vi "FR GUI Measurement setup.vi"(7 "Common properties":T1={"Measurement status ref"=refnum, "TWM Status ref"=refnum, "Abort ref"=refnum, "Skip waiting ref"=refnum, "GNU Octave path"=path "C:/Program Files/GNU Octave/Octave-6.2.0/mingw64/bin", "TWM+QWTB path"=path "C:/Users/labina/Desktop/TWM-1.8.7.0-full/octprog", "lvlib path"=path "D:/martin/WAC/WACsw - github/control_software/Filter function meter/external libraries/GOLPI 0.7.3.1 source distribution LV 20.0 32 bit/lv_proc.dll", "TWM pipe"="\\\\.\\pipe\\TWM:server", "PJVS status ref"=refnum, "WAC path"=path ""}, 8 "DC meter":T2={"DC meter type"=enum."H/A/K 3458", "DC meter VISA"="", "NPLC"=10.0, "status ref"=refnum}, 9 "FR measurement":T4={"Measurement frequencies (Hz)"=[1000.0, 10000.0, 1000.0], "Sampling frequency (Hz)"=500000.0, "Signal amplitude (V)"=4.5, "AC-DC settle time (s)"=20.0, "Record length (multiples of period)"=[1000.0, 10000.0, 1000.0], "Measurement template file"=path "", "Row of START keyword"=0, "Row of STOP keyword"=0, "Calculate RMS from samples"=FALSE, "AC-DC warm up time (s)"=300.0, "Measurement template line"=[], "DC meter readings No."=10, "Algorithm"="TWM-WFFT", "Simultaneous measurement"=FALSE, "Recalculate-skip already calculated"=FALSE} {"Record length (multiples of period)" format="%#_3p"; "Sampling frequency (Hz)" format="%#_3p"; "Measurement frequencies (Hz)" format="%#_3p"}) -> (1 "Common properties out":T1={"Measurement status ref"=refnum, "TWM Status ref"=refnum, "Abort ref"=refnum, "Skip waiting ref"=refnum, "GNU Octave path"=path "C:/Program Files/GNU Octave/Octave-6.2.0/mingw64/bin", "TWM+QWTB path"=path "C:/Users/labina/Desktop/TWM-1.8.7.0-full/octprog", "lvlib path"=path "D:/martin/WAC/WACsw - github/control_software/Filter function meter/external libraries/GOLPI 0.7.3.1 source distribution LV 20.0 32 bit/lv_proc.dll", "TWM pipe"="\\\\.\\pipe\\TWM:server", "PJVS status ref"=refnum, "WAC path"=path ""}, 3 "FR measurement out":T4={"Measurement frequencies (Hz)"=[1000.0, 10000.0, 1000.0], "Sampling frequency (Hz)"=500000.0, "Signal amplitude (V)"=4.5, "AC-DC settle time (s)"=20.0, "Record length (multiples of period)"=[1000.0, 10000.0, 1000.0], "Measurement template file"=path "", "Row of START keyword"=0, "Row of STOP keyword"=0, "Calculate RMS from samples"=FALSE, "AC-DC warm up time (s)"=300.0, "Measurement template line"=[], "DC meter readings No."=10, "Algorithm"="TWM-WFFT", "Simultaneous measurement"=FALSE, "Recalculate-skip already calculated"=FALSE} {"Record length (multiples of period)" format="%#_3p"; "Sampling frequency (Hz)" format="%#_3p"; "Measurement frequencies (Hz)" format="%#_3p"})   [LabVIEW 2020]
doc: "GUI to setup parameters of the mesurement procedure used to estimate frequency response of the digitizer."
uses:
  FR Measurement/Type definitions/FR measuement.ctl
  General DC meter/Type definitions/DC meter.ctl
  General DC meter/Type definitions/DC meter type.ctl
  Utilities/Type definitions/Common properties.ctl
  <vilib>/Utility/error.llb/Error Cluster From Error Code.vi
  <vilib>/ErrorRing/Error Ring.xnode
  external libraries/varilib/varilib.lvlib
panel:
  out "Simultaneous\nmeasurement":bool
  out "Algorithm":string
  out "dc meter readings":i32=50000 caption="DC meter readings"
  in  "recalculate template":bool
  out "ac-dc warmup time":dbl=50000.0 caption="AC-DC warm-up time" format="%#_6p"
  out "Estimate as formatted text":string
  out "Meas points":i32=1 caption="Measurement points"
  in  "Calculate RMS\nfrom samples":bool
  out "ac-dc settle time":dbl=50000.0 caption="AC-DC settle time" format="%#_6p"
  out "Measurement freq. (Hz) | Record length (periods)":dbl[][](array[numeric])=[[1000.0]] format="%#_3p"
  in  "load template":bool
  in  "Measurement template file":path
  in  "show connections":bool
  out "Signal amplitude (V)":dbl=1.0 caption="AC voltage amplitude"
  out "Sampling frequency (Hz)":dbl=50000.0 caption="Sampling frequency" format="%#_6p"
  out "gui_elements":refnum<vi>[](array[refnum])
  in  "save_and_quit":bool
  in  "cancel":bool
  # "Load the template and check loaded values here:"
  # "s"
  # "V"
  # "Who will make\nnice pictures?\n\nconnection setup here"
  # "Hz"
  # "s"
  # "Who will make\nnice pictures?\n\nwaveforms here"
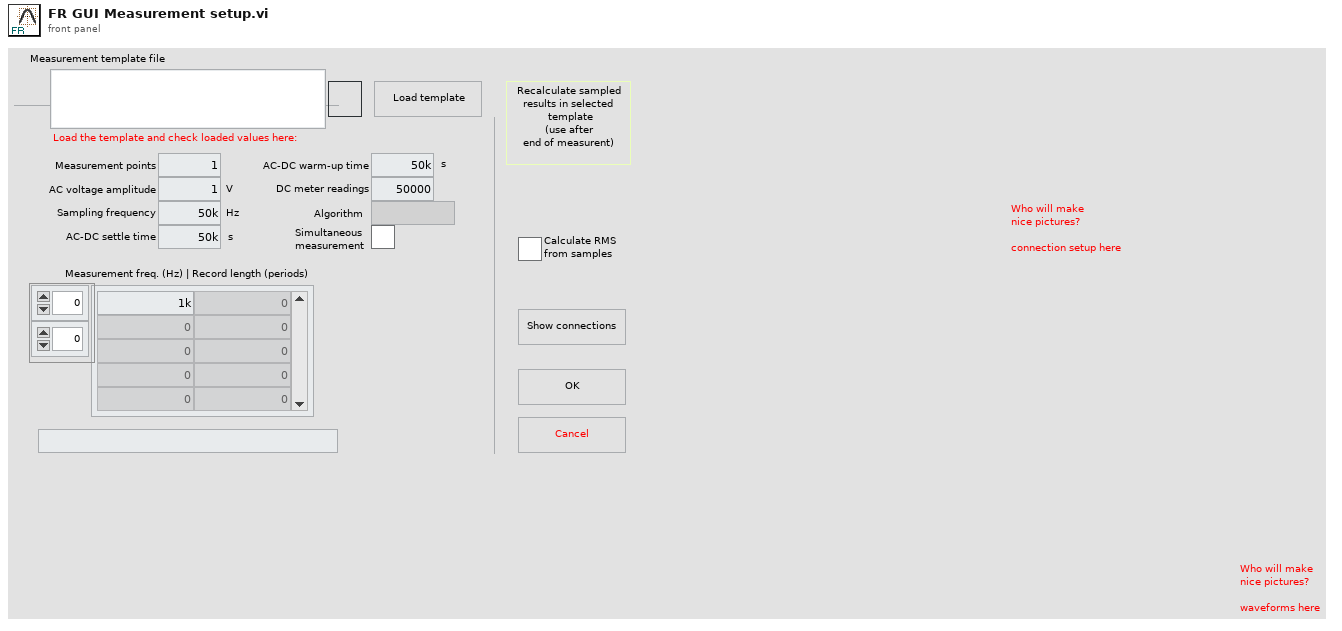
[diagram p1: front panel]
types:
  T1 = typedef "Common properties.ctl" = cluster{"Measurement status ref":refnum<vi>, "TWM Status ref":refnum<vi>, "Abort ref":refnum<vi>, "Skip waiting ref":refnum<vi>, "GNU Octave path":path, "TWM+QWTB path":path, "lvlib path":path, "TWM pipe":string, "PJVS status ref":refnum<vi>, "WAC path":path}
  T2 = typedef "DC meter.ctl" = cluster{"DC meter type":T3, "DC meter VISA":refnum<visa-resource-name>, "NPLC":dbl, "status ref":refnum<vi>}
  T3 = typedef "DC meter type.ctl" = enum16{"H/A/K 3458", "Fluke 8508A", "dummy", "Keithley 2182"}
  T4 = typedef "FR measuement.ctl" = cluster{"Measurement frequencies (Hz)":dbl[], "Sampling frequency (Hz)":dbl, "Signal amplitude (V)":dbl, "AC-DC settle time (s)":dbl, "Record length (multiples of period)":dbl[], "Measurement template file":path, "Row of START keyword":i32, "Row of STOP keyword":i32, "Calculate RMS from samples":bool, "AC-DC warm up time (s)":dbl, "Measurement template line":i32[], "DC meter readings No.":i32, "Algorithm":string, "Simultaneous measurement":bool, "Recalculate-skip already calculated":bool}
  T5 = enum32{"Bad", "Idle", "Run top level", "Running"}
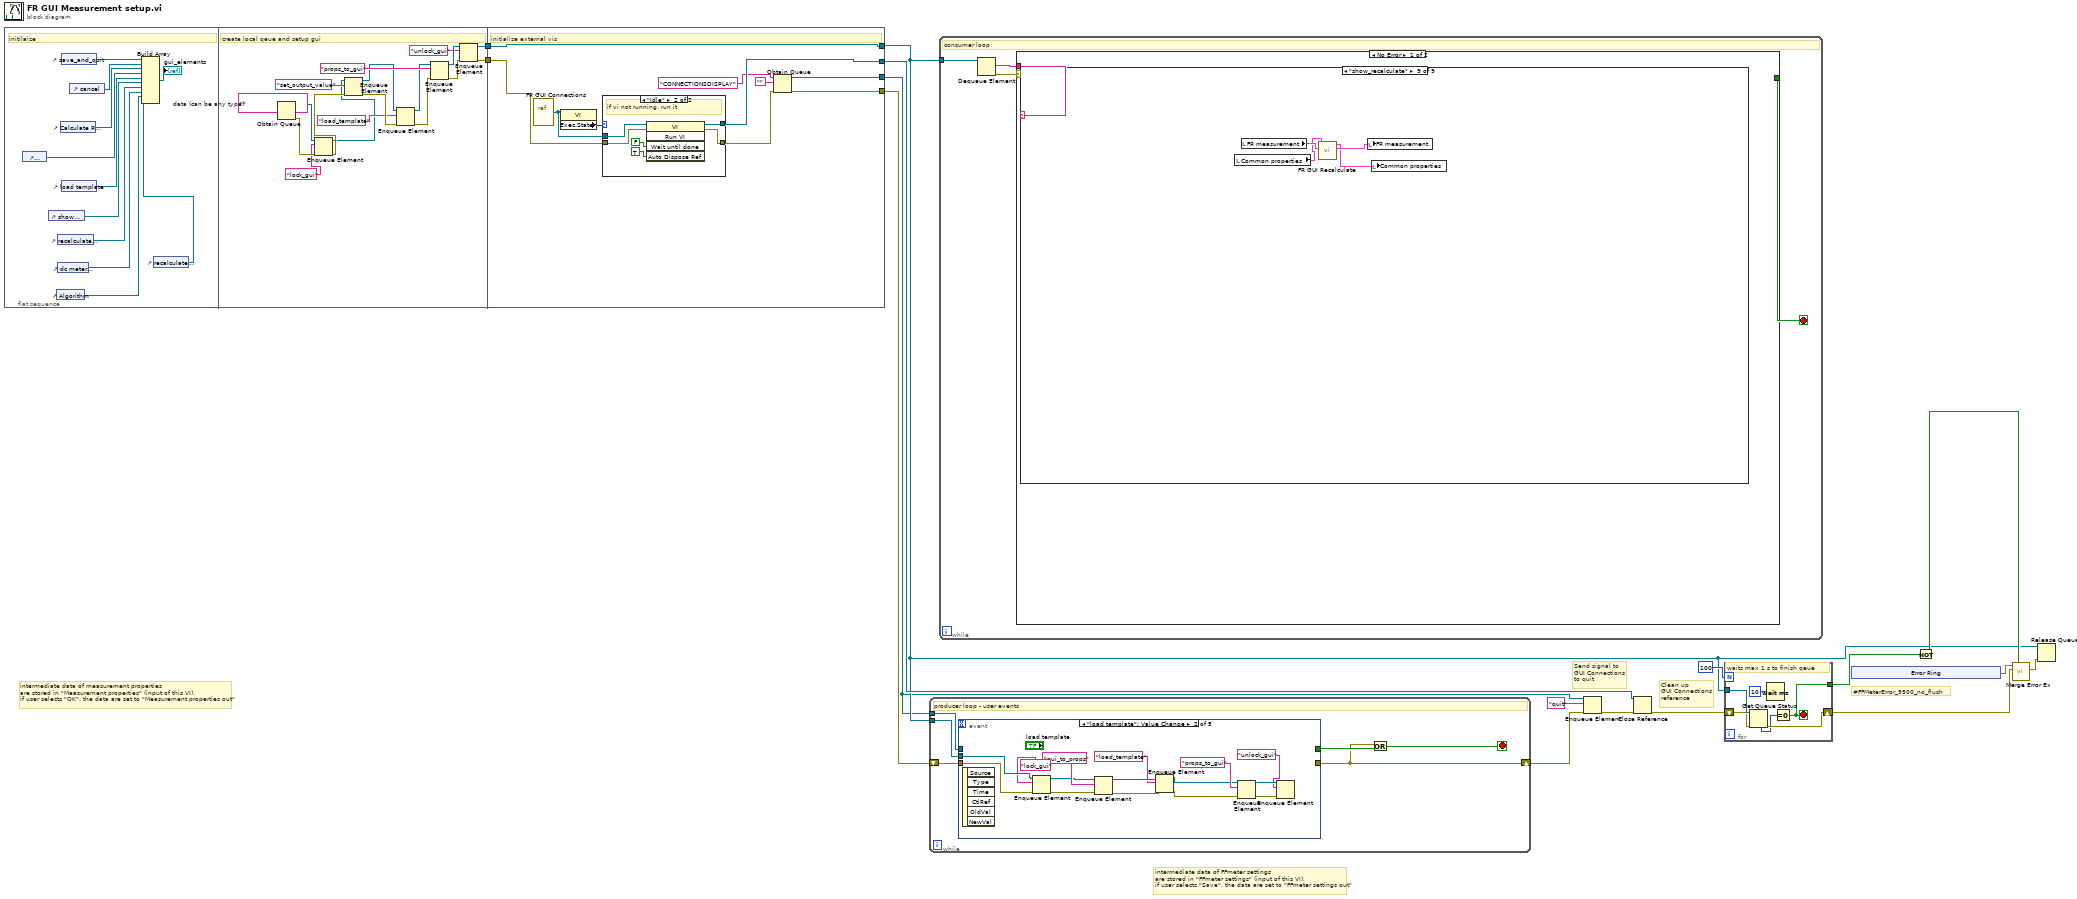
[diagram p0: block diagram]
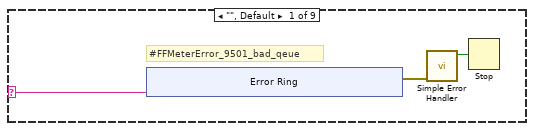
[diagram p3: hidden frame]
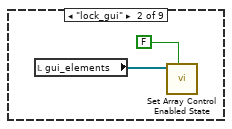
[diagram p4: hidden frame]
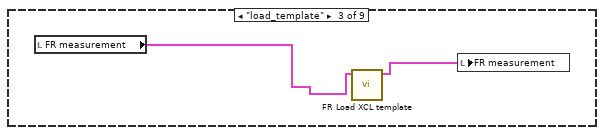
[diagram p5: hidden frame]
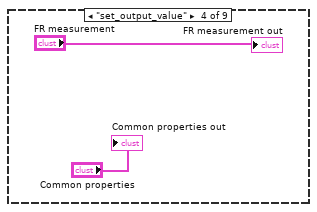
[diagram p6: hidden frame]
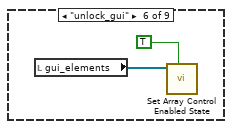
[diagram p8: hidden frame]
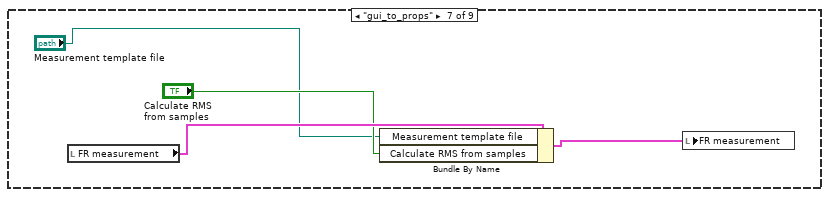
[diagram p9: hidden frame]
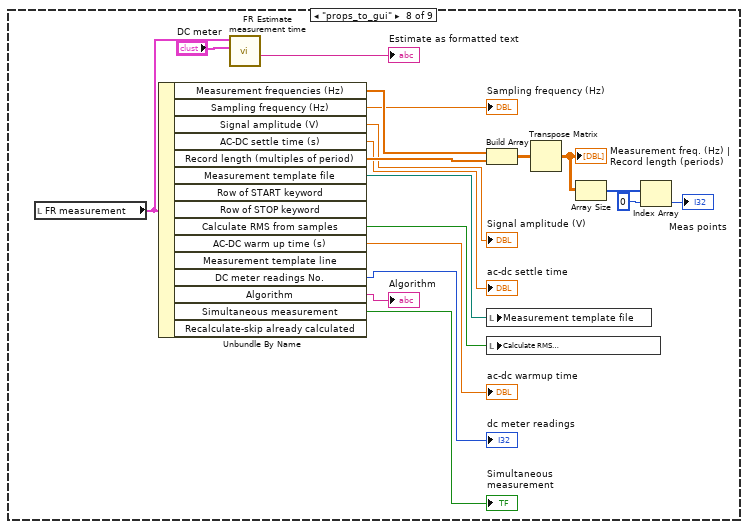
[diagram p10: hidden frame]
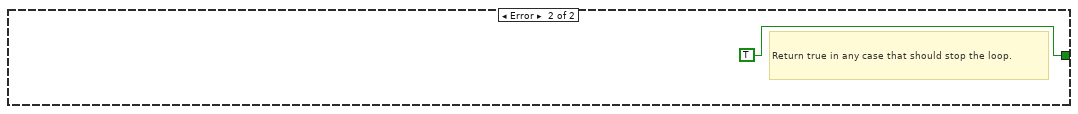
[diagram p11: hidden frame]
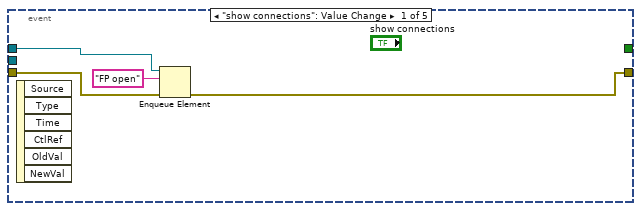
[diagram p12: hidden frame]
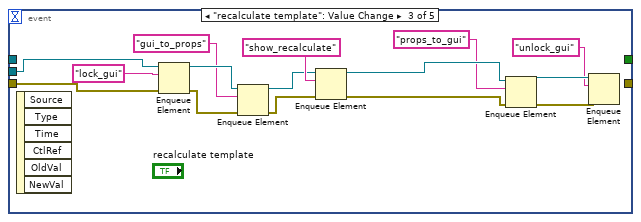
[diagram p13: hidden frame]
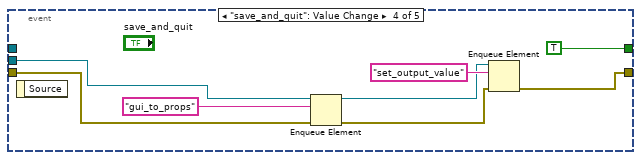
[diagram p14: hidden frame]
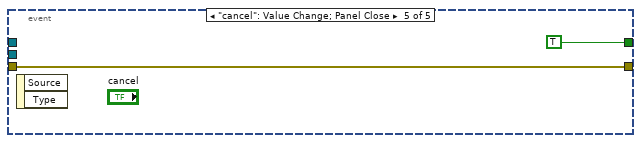
[diagram p15: hidden frame]
diagram:
  # "intermediate data of measurement properties\nare stored in \"Measurement properties\" (input of this VI),\nif user selects \"OK\", the data are set to \"Measurement properties out\""
  # "intermediate data of FFmeter settings\nare stored in \"FFmeter settings\" (input of this VI),\nif user selects \"Save\", the data are set to \"FFmeter settings out\""
  # "Send signal to\nGUI Connections\nto quit"
  # "Clean up\nGUI Connections\nreference"
  # "#FFMeterError_9500_no_flush"
  n1 = flat-sequence {
    tunnel: [w41] -> w9
    tunnel: [w42] -> w8
    tunnel: [w51] -> w10
    tunnel: [w55] -> w3
    tunnel: w9 -> [w55]
    tunnel: w8 -> [w54]
    tunnel: [w52] -> w2
    tunnel: [w53] -> w5
    frame #0 {
      # "initilaize"
      n2 = control-ref of="Measurement template file"() -> (w23:refnum<vi>)
      n3 = control-ref of="show connections"() -> (w21:refnum<vi>)
      n4 = control-ref of="Algorithm"() -> (w18:refnum<vi>)
      n5 = control-ref of="dc meter readings"() -> (w19:refnum<vi>)
      n6 = control-ref of="recalculate template"() -> (w20:refnum<vi>)
      n7 = control-ref of="Calculate RMS\nfrom samples"() -> (w24:refnum<vi>)
      n8 = control-ref of="save_and_quit"() -> (w27:refnum<vi>)
      n9 = control-ref of="load template"() -> (w22:refnum<vi>)
      n10 = control-ref of="cancel"() -> (w26:refnum<vi>)
      n11 = control-ref of="recalculate template"() -> (w17:refnum<vi>)
      n12 = Build Array(w27, w26, w24, w23, w22, w21, w20, w19, w18, w17) -> (→"gui_elements":refnum<vi>[])
    }
    frame #1 {
      w44 = ""  # data (can be any type)
      # "create local qeue and setup gui"
      n13 = Obtain Queue(element data type=w44) -> (queue out=w29:refnum<queue>, error out=w32:errorcluster)  [unwired: 4 in, 1 out]
      n14 = Enqueue Element(queue=w29, element="lock_gui", error in (no error)=w32) -> (queue out=w30:refnum<queue>, error out=w31:errorcluster)  [unwired: 1 in, 1 out]
      n15 = Enqueue Element(queue=w30, element="set_output_value", error in (no error)=w31) -> (queue out=w35:refnum<queue>, error out=w37:errorcluster)  [unwired: 1 in, 1 out]
      n16 = Enqueue Element(queue=w35, element="load_template", error in (no error)=w37) -> (queue out=w34:refnum<queue>, error out=w36:errorcluster)  [unwired: 1 in, 1 out]
      n17 = Enqueue Element(queue=w34, element="props_to_gui", error in (no error)=w36) -> (queue out=w40:refnum<queue>, error out=w43:errorcluster)  [unwired: 1 in, 1 out]
      n18 = Enqueue Element(queue=w40, element="unlock_gui", error in (no error)=w43) -> (queue out=w41:refnum<queue>, error out=w42:errorcluster)  [unwired: 1 in, 1 out]
    }
    frame #2 {
      # "initialize external vis"
      n19 = vi-ref "FR GUI Connections.vi"() -> (w49:refnum<vi>)
      n20 = property class="VI"(reference=w49) -> ("Exec.State"=w50:T5)  [unwired: 1 in, 2 out]
      n21 = case shown="\"Idle\"" w50 {
        tunnel: [w56 w63] -> w46
        tunnel: w54 -> [w56 w60]
        tunnel: [w57 w59] -> w53
        tunnel: w49 -> [w57 w58]
        frame "Bad", Default {
        }
        frame "Idle" {
          # "if vi not running, run it"
          n22 = invoke class="VI" method="Run VI"(reference=w58, error in=w60, "Wait until done"=FALSE ("Wait Until Done"), "Auto Dispose Ref"=TRUE ("Wait Until Done")) -> (reference out=w59:refnum<vi>, error out=w63:errorcluster)  [unwired: 1 in, 3 out]
        }
      }
      n23 = Obtain Queue(name (unnamed)="CONNECTIONSDISPLAY", element data type="", error in (no error)=w46) -> (queue out=w52:refnum<queue>, error out=w51:errorcluster)  [unwired: 2 in, 1 out]
    }
  }
  n24 = while {
    shift-right: [w65] -> w4
    shift-left: w10 -> [w68]
    tunnel: w3 -> [w69]
    tunnel: w2 -> [w64]
    stop <- w66 stop-if-true
    # "producer loop - user events"
    n25 = event shown="[1] \"load template\": Value Change" {
      selector: _ -> [_ _ _ _ _]
      dyn-events: _ -> [_ _ _ _ _]
      timeout: _ -> [_ _ _ _ _]
      tunnel: w69 -> [_ w78 w98 w110 _]
      tunnel: w68 -> [w72 w75 w99 w109 w112]
      tunnel: [w71 _ _ w107 w112] -> w65
      tunnel: [_ _ _ TRUE ("cancel") TRUE ("cancel")] -> w67
      tunnel: w64 -> [w70 _ _ _ _]
      event "show connections": Value Change {
        n26 = event-data() -> ()  [unwired: 1 in, 6 out]
        n27 = Enqueue Element(queue=w70, element="FP open", error in (no error)=w72) -> (error out=w71:errorcluster)  [unwired: 1 in, 2 out]
      }
      event "load template": Value Change {
        n28 = event-data() -> ()  [unwired: 1 in, 6 out]
        n29 = Enqueue Element(queue=w78, element="lock_gui", error in (no error)=w75) -> (queue out=w77:refnum<queue>, error out=w76:errorcluster)  [unwired: 1 in, 1 out]
        n30 = Enqueue Element(queue=w77, element="gui_to_props", error in (no error)=w76) -> (queue out=w84:refnum<queue>, error out=w86:errorcluster)  [unwired: 1 in, 1 out]
        n31 = Enqueue Element(queue=w84, element="load_template", error in (no error)=w86) -> (queue out=w83:refnum<queue>, error out=w85:errorcluster)  [unwired: 1 in, 1 out]
        n32 = Enqueue Element(queue=w83, element="props_to_gui", error in (no error)=w85) -> (queue out=w80:refnum<queue>, error out=w81:errorcluster)  [unwired: 1 in, 1 out]
        n33 = Enqueue Element(queue=w80, element="unlock_gui", error in (no error)=w81) -> ()  [unwired: 1 in, 3 out]
      }
      event "recalculate template": Value Change {
        n34 = event-data() -> ()  [unwired: 1 in, 6 out]
        n35 = Enqueue Element(queue=w98, element="lock_gui", error in (no error)=w99) -> (queue out=w93:refnum<queue>, error out=w96:errorcluster)  [unwired: 1 in, 1 out]
        n36 = Enqueue Element(queue=w93, element="gui_to_props", error in (no error)=w96) -> (queue out=w94:refnum<queue>, error out=w95:errorcluster)  [unwired: 1 in, 1 out]
        n37 = Enqueue Element(queue=w94, element="show_recalculate", error in (no error)=w95) -> (queue out=w101:refnum<queue>, error out=w102:errorcluster)  [unwired: 1 in, 1 out]
        n38 = Enqueue Element(queue=w101, element="props_to_gui", error in (no error)=w102) -> (queue out=w90:refnum<queue>, error out=w91:errorcluster)  [unwired: 1 in, 1 out]
        n39 = Enqueue Element(queue=w90, element="unlock_gui", error in (no error)=w91) -> ()  [unwired: 1 in, 3 out]
      }
      event "save_and_quit": Value Change {
        n40 = event-data() -> ()  [unwired: 1 in, 1 out]
        n41 = Enqueue Element(queue=w110, element="gui_to_props", error in (no error)=w109) -> (queue out=w104:refnum<queue>, error out=w108:errorcluster)  [unwired: 1 in, 1 out]
        n42 = Enqueue Element(queue=w104, element="set_output_value", error in (no error)=w108) -> (error out=w107:errorcluster)  [unwired: 1 in, 2 out]
      }
      event "cancel": Value Change; Panel Close {
        n43 = event-data() -> ()  [unwired: 1 in, 2 out]
      }
    }
    n44 = Or(x=w65, y=w67) -> (x .or. y?=w66:bool)
  }
  n45 = while {
    tunnel: w3 -> [w117]
    stop <- w114 stop-if-true
    # "consumer loop"
    n46 = Dequeue Element(queue=w117) -> (element=w115:string, error out=w116:errorcluster)  [unwired: 2 in, 2 out]
    n47 = case shown="No Error" w116 {
      tunnel: w115 -> [w118 _]
      tunnel: [_ TRUE] -> w114
      frame No Error {
        n48 = case shown="\"show_recalculate\"" w118 {
          selector: w118 -> [w119 _ _ _ _ _ _ _ _]
          frame "", Default {
            # "#FFMeterError_9501_bad_qeue"
            n49 = xnode "Error Ring"("parameter 0"=w119) -> ("error out"=w121:errorcluster)
            n50 = call <vilib>:"Simple Error Handler.vi"("error in (no error)"=w121) -> ("error?"=w120:bool)  [unwired: 4 in, 4 out]
            n51 = Stop(stop? (T)=w120) -> ()
          }
          frame "lock_gui" {
            n52 = local read "gui_elements"() -> (w130:refnum<vi>[])
            n53 = call "Set Array Control Enabled State.vi"("enabled (T)"=FALSE, "reference array in"=w130) -> ()  [unwired: 8 in, 2 out]
          }
          frame "load_template" {
            n54 = local read "FR measurement"() -> (w131:T4)
            n55 = call "FR Load XCL template.vi"("FR measurement"=w131) -> ("FR measurement out"=w132:T4)  [unwired: 10 in]
            n56 = local write "FR measurement"(w132) -> ()
          }
          frame "set_output_value" {
            "FR measurement out" <- "FR measurement"
            "Common properties out" <- "Common properties"
          }
          frame "create_template" {
          }
          frame "unlock_gui" {
            n57 = local read "gui_elements"() -> (w136:refnum<vi>[])
            n58 = call "Set Array Control Enabled State.vi"("enabled (T)"=TRUE, "reference array in"=w136) -> ()  [unwired: 8 in, 2 out]
          }
          frame "gui_to_props" {
            n59 = local read "FR measurement"() -> (w140:T4)
            n60 = Bundle By Name(cluster=w140, "Measurement template file"="Measurement template file", "Calculate RMS from samples"="Calculate RMS\nfrom samples") -> (w138:T4)
            n61 = local write "FR measurement"(w138) -> ()
          }
          frame "props_to_gui" {
            n62 = local read "FR measurement"() -> (w142:T4)
            n63 = Unbundle By Name(w142) -> ("Measurement frequencies (Hz)"=w153:dbl[], "Sampling frequency (Hz)"=→"Sampling frequency (Hz)":dbl, "Signal amplitude (V)"=→"Signal amplitude (V)":dbl, "AC-DC settle time (s)"=→"ac-dc settle time":dbl, "Record length (multiples of period)"=w152:dbl[], "Measurement template file"=w148:path, "Calculate RMS from samples"=w147:bool, "AC-DC warm up time (s)"=→"ac-dc warmup time":dbl, "DC meter readings No."=→"dc meter readings":i32, "Algorithm"=→"Algorithm":string, "Simultaneous measurement"=→"Simultaneous\nmeasurement":bool)  [unwired: 4 out]
            n64 = call "FR Estimate measurement time.vi"("DC meter"="DC meter", "FR measurement"=w142) -> ("Estimate as formatted text"=→"Estimate as formatted text":string)  [unwired: 8 in, 1 out]
            n65 = Build Array(w153, w152) -> (w159:dbl[][])
            n66 = local write "Measurement template file"(w148) -> ()
            n67 = local write "Calculate RMS\nfrom samples"(w147) -> ()
            n68 = Transpose Matrix(1:w159) -> (0:w158:dbl[][])
            "Measurement freq. (Hz) | Record length (periods)" <- w158
            n69 = Array Size(array=w158) -> (size(s)=w157:i32[])
            n70 = Index Array(array=w157, index=0) -> (element=→"Meas points":i32)
          }
          frame "show_recalculate" {
            n71 = local read "Common properties"() -> (w160:T1)
            n72 = local read "FR measurement"() -> (w163:T4)
            n73 = call "FR GUI Recalculate.vi"("FR measurement"=w163, "Common properties"=w160) -> ("FR measurement out"=w162:T4, "Common properties out"=w161:T1)  [unwired: 8 in]
            n74 = local write "FR measurement"(w162) -> ()
            n75 = local write "Common properties"(w161) -> ()
          }
        }
      }
      frame Error {
        # "Return true in any case that should stop the loop."
      }
    }
  }
  n76 = Enqueue Element(queue=w2, element="quit", error in (no error)=w4) -> (error out=w7:errorcluster)  [unwired: 1 in, 2 out]
  n77 = Close Reference(reference=w5, error in (no error)=w7) -> (error out=w1:errorcluster)
  n78 = for {
    N: 100 -> [_]
    tunnel: w3 -> [w170]
    shift-right: [w168] -> w13
    shift-left: w1 -> [w169]
    tunnel: [w165] -> w11
    stop <- w165 stop-if-true
    # "waits max 1 s to finish qeue"
    n79 = Get Queue Status(queue=w170, error in (no error)=w169) -> (error out=w168:errorcluster, # elements in queue=w166:i32)  [unwired: 1 in, 6 out]
    n80 = Wait (ms)(milliseconds to wait=u32 10) -> ()  [unwired: 1 out]
    n81 = Equal To 0?(x=w166) -> (x = 0?=w165:bool)
  }
  n82 = xnode "Error Ring"() -> ("error out"=w14:errorcluster)
  n83 = Not(x=w11) -> (.not. x?=w15:bool)
  n84 = call "Merge Error Ex.vi"("Is error? (False)"=w15, "main error in (no error)"=w13, "second error in"=w14) -> ("error out"=w12:errorcluster)  [unwired: 8 in]
  n85 = Release Queue(queue=w3, error in (no error)=w12) -> ()  [unwired: 1 in, 3 out]
